vi "1.5主程序.vi"() -> ()   [LabVIEW 2016]
panel:
  out "test_answer":dbl
  in  "test_value2":dbl
  in  "test_value1":dbl
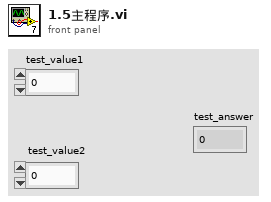
[diagram p1: front panel]
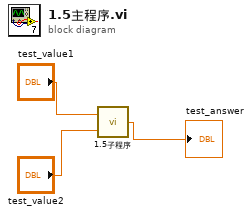
[diagram p0: block diagram]
diagram:
  n1 = call "1.5子程序.vi"("value2"="test_value2", "value1"="test_value1") -> ("max_value"=→"test_answer":dbl)
